vi "SSC Digital Calculate Per-Site Per-Pin to Per-Instrument LUT.vi"(0 "Digital SSC In":T2[](array[typedef]), 7 "Sites":i32[](array[numeric]), 9 "Pins":tag[](array[tag])) -> (4 "Per-Site Per-Pin to Per-Instrument LUT":T1[][](array[typedef]), 6 "Instrument Count":i32, 8 "Max Sites on Instrument":i32)   [LabVIEW 2019]
uses:
  SSC Digital/SSC Digital.ctl
  Digital 2D Location.ctl
  Shared SubVIs/Trim Whitespace [Inlined].vi
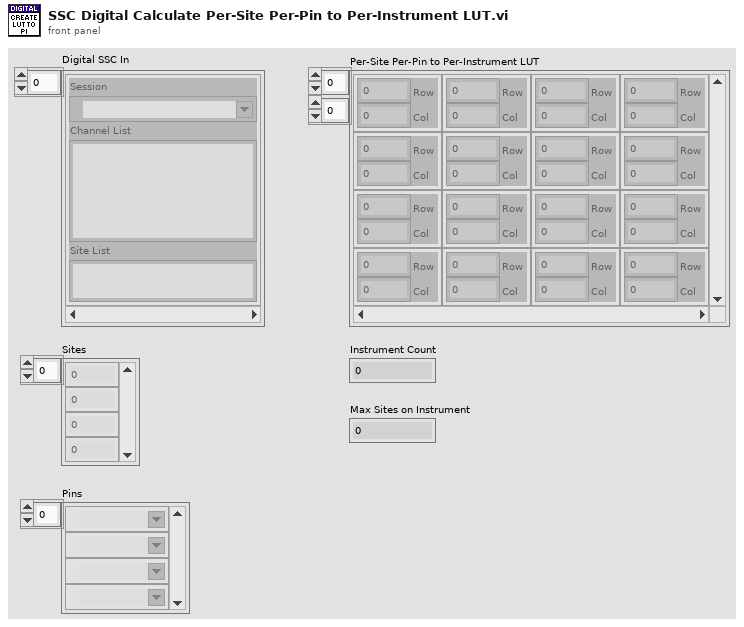
[diagram p1: front panel]
types:
  T1 = typedef "Digital 2D Location.ctl" = cluster{"Row":i32, "Col":i32}
  T2 = typedef "SSC Digital.ctl" = cluster{"Session":refnum<k15>, "Channel List":string, "Site List":string}
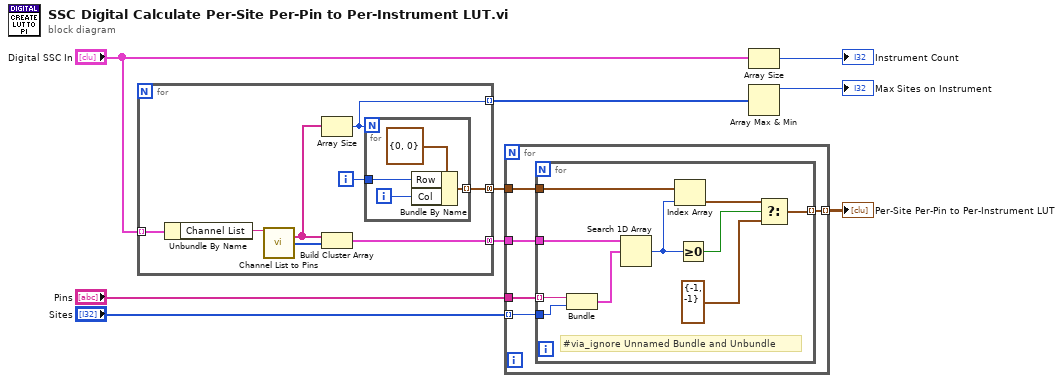
[diagram p0: block diagram]
diagram:
  n1 = for {
    tunnel: "Digital SSC In" -> [w17] mode=indexing
    tunnel: [w14] -> w6 mode=concatenating
    tunnel: [w11] -> w5 mode=concatenating
    tunnel: [w10] -> w2 mode=indexing
    i -> [w12]
    n2 = Unbundle By Name(w17) -> ("Channel List"=w16:string)
    n3 = call "Channel List to Pins.vi"("Channel List"=w16) -> ("Pins"=w13:tag[], "Sites"=w15:i32[])  [unwired: 12 in, 1 out]
    n4 = Array Size(array=w13) -> (size(s)=w10:i32)
    n5 = Build Cluster Array(w13, w15) -> (w14:cluster{"Pin":tag, "trimmed string":i32}[])
    n6 = for {
      N: w10 -> [_]
      tunnel: w12 -> [w19]
      tunnel: [w20] -> w11 mode=indexing
      i -> [w18]
      n7 = Bundle By Name(cluster=T1 {"Row"=0, "Col"=0}, "Row"=w19, "Col"=w18) -> (w20:T1)
    }
  }
  n8 = for {
    tunnel: "Sites" -> [w24] mode=indexing
    tunnel: "Pins" -> [w25]
    tunnel: [w26] -> w7 mode=indexing
    tunnel: w6 -> [w23]
    tunnel: w5 -> [w22]
    n9 = for {
      tunnel: [w30] -> w26 mode=indexing
      tunnel: w25 -> [w35] mode=indexing
      tunnel: w24 -> [w34]
      tunnel: w23 -> [w36]
      tunnel: w22 -> [w32]
      # "#via_ignore Unnamed Bundle and Unbundle"
      n10 = Bundle("Pin"=w35, "Site Number"=w34) -> (w33:cluster{"Pin":tag, "Site Number":i32})  [unwired: 1 in]
      n11 = Search 1D Array(1D array=w36, element=w33) -> (index of element=w29:i32)  [unwired: 1 in]
      n12 = Index Array(array=w32, index=w29) -> (element=w31:T1)
      n13 = Greater Or Equal To 0?(x=w29) -> (x >= 0?=w28:bool)
      n14 = Select(t=w31, s=w28, f=T1 {"Row"=-1, "Col"=-1}) -> (s? t:f=w30:T1)
    }
  }
  "Per-Site Per-Pin to Per-Instrument LUT" <- w7
  n15 = Array Size(array="Digital SSC In") -> (size(s)=→"Instrument Count":i32)
  n16 = Array Max & Min(array=w2) -> (max value=→"Max Sites on Instrument":i32)  [unwired: 3 out]
